vi "GV gating.vi"() -> ()   [LabVIEW 2017]
panel:
  out "Gating":bool
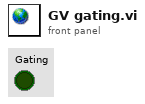
[diagram p1: front panel]
diagram:
